vi "Construct_Log_File_Path.vi"(8 "error in (no error)":errorcluster, 10 "filename without extension":string, 11 "build":refnum<class "AB_Build.lvclass">) -> (0 "error out":errorcluster, 3 "appended path":path)   [LabVIEW 2020, in "AB_Build.lvclass"]
uses:
  <vilib>/AppBuilder/AB_Classes/Build/AB_Build.lvclass
  <vilib>/AppBuilder/AB_Classes/Build/AB_Build.lvclass/AB_Build.ctl
  <vilib>/AppBuilder/AB_Classes/Destination/AB_Destination.lvclass
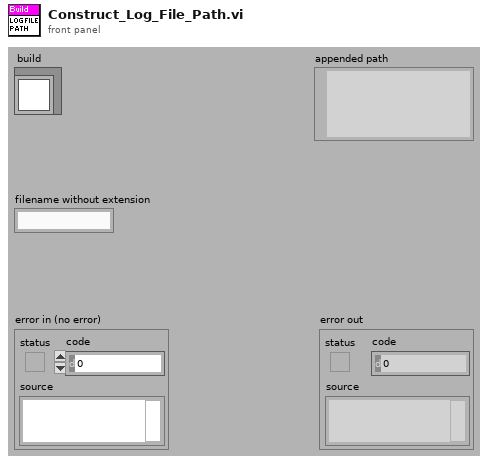
[diagram p1: front panel]
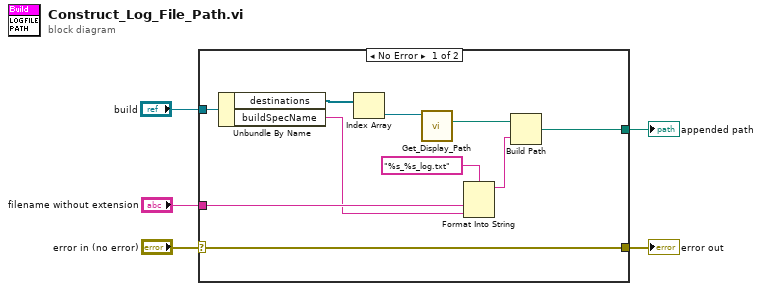
[diagram p0: block diagram]
diagram:
  n1 = case shown="No Error" "error in (no error)" {
    selector: "error in (no error)" -> [w7 w16]
    tunnel: "filename without extension" -> [w15 _]
    tunnel: [w9 _] -> w4
    tunnel: [w7 w16] -> w2
    tunnel: "build" -> [w6 _]
    frame No Error {
      n2 = Unbundle By Name(w6) -> ("destinations"=w8:refnum<class "AB_Destination.lvclass">[], "buildSpecName"=w12:string)
      n3 = Index Array(array=w8) -> (element=w13:refnum<class "AB_Destination.lvclass">)  [unwired: 1 in]
      n4 = call-dynamic "Get_Display_Path.vi"("AB_Destination in"=w13) -> ("displayPath"=w14:path)  [unwired: 1 in, 9 out]
      n5 = Format Into String(format string="%s_%s_log.txt", w15, w12) -> (resulting string=w11:string)  [unwired: 2 in, 1 out]
      n6 = Build Path(base path=w14, name or relative path=w11) -> (appended path=w9:path)
    }
    frame Error {
    }
  }
  "appended path" <- w4
  "error out" <- w2
